vi "Check Resize.vi"(8 "error in (no error)":errorcluster, 11 "HistorianCharting in":refnum<class "HistorianCharting.lvclass">) -> (0 "error out":errorcluster, 3 "HistorianCharting out":refnum<class "HistorianCharting.lvclass">)   [LabVIEW 2020, in "VolatusGUIElements.lvlib" / "HistorianCharting.lvclass"]
uses:
  HistorianCharting.lvclass
  HistorianCharting.lvclass/HistorianCharting.ctl
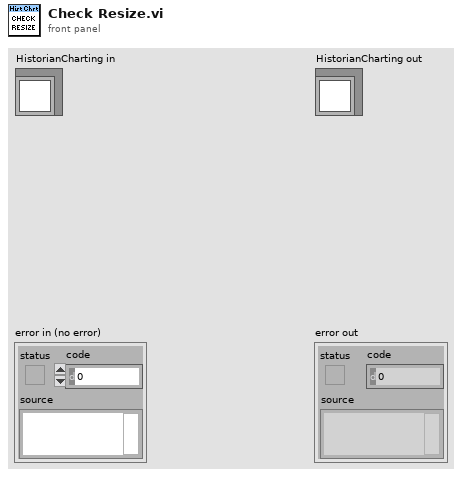
[diagram p1: front panel]
types:
  T1 = typedef "LVBoundsTypeDef.ctl" = cluster{"Width":u32, "Height":u32}
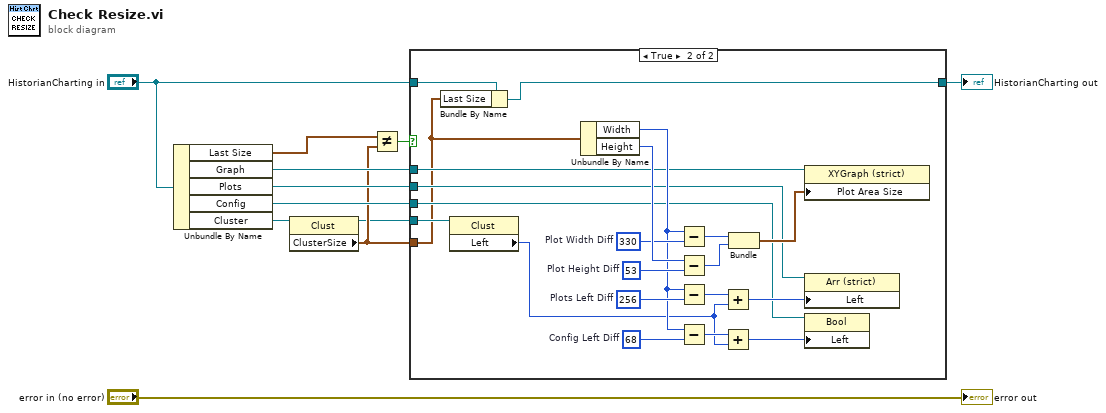
[diagram p0: block diagram]
diagram:
  n1 = Unbundle By Name("HistorianCharting in") -> ("Last Size"=w9:T1, "Graph"=w3:refnum<vi>, "Plots"=w4:refnum<vi>, "Config"=w5:refnum<vi>, "Cluster"=w10:refnum<vi>)
  n2 = property class="Clust"(reference=w10) -> (reference out=w1:refnum<vi>, "ClusterSize"=w2:T1)  [unwired: 1 in, 1 out]
  n3 = Not Equal?(x=w9, y=w2) -> (x != y?=w7:bool)
  n4 = case shown="True" w7 {
    tunnel: "HistorianCharting in" -> [w12 w33]
    tunnel: [w12 w32] -> w6
    tunnel: w5 -> [_ w15]
    tunnel: w4 -> [_ w17]
    tunnel: w3 -> [_ w19]
    tunnel: w2 -> [_ w13]
    tunnel: w1 -> [_ w31]
    frame False {
    }
    frame True {
      w28 = u32 53  # Plot Height Diff
      w29 = u32 330  # Plot Width Diff
      w23 = u32 68  # Config Left Diff
      w25 = u32 256  # Plots Left Diff
      n5 = Bundle By Name(cluster=w33, "Last Size"=w13) -> (w32:refnum<class "HistorianCharting.lvclass">)
      n6 = property class="Clust"(reference=w31) -> ("Left"=w20:i32)  [unwired: 1 in, 2 out]
      n7 = Unbundle By Name(w13) -> ("Width"=w24:u32, "Height"=w30:u32)
      n8 = Subtract(x=w24, y=w29) -> (x-y=w27:u32)
      n9 = Subtract(x=w30, y=w28) -> (x-y=w26:u32)
      n10 = Subtract(x=w24, y=w25) -> (x-y=w22:u32)
      n11 = Subtract(x=w24, y=w23) -> (x-y=w21:u32)
      n12 = Add(x=w22, y=w20) -> (x+y=w16:u32)
      n13 = Add(x=w21, y=w20) -> (x+y=w14:u32)
      n14 = Bundle(w27, w26) -> (w18:cluster{u32, u32})  [unwired: 1 in]
      n15 = property class="XYGraph (strict)"(reference=w19, "Plot Area Size"=w18) -> ()  [unwired: 1 in, 2 out]
      n16 = property class="Arr (strict)"(reference=w17, "Left"=w16) -> ()  [unwired: 1 in, 2 out]
      n17 = property class="Bool"(reference=w15, "Left"=w14) -> ()  [unwired: 1 in, 2 out]
    }
  }
  "HistorianCharting out" <- w6
  "error out" <- "error in (no error)"
